vi "write_attributes.vi"(8 "error in (no error)":errorcluster, 10 "attributes":T1, 11 "LinearSVC in":refnum<class "LinearSVC.lvclass">) -> (0 "error out":errorcluster, 3 "LinearSVC out":refnum<class "LinearSVC.lvclass">)   [LabVIEW 2020, in "LinearSVC.lvclass"]
uses:
  LinearSVC.lvclass
  Controls/linear_svc_attributes.ctl
  LinearSVC.lvclass/LinearSVC.ctl
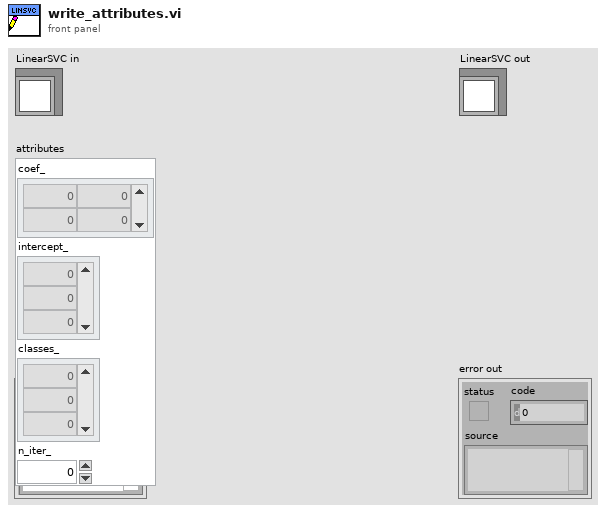
[diagram p1: front panel]
types:
  T1 = typedef "linear_svc_attributes.ctl" = cluster{"coef_":dbl[][], "intercept_":dbl[], "classes_":dbl[], "n_iter_":dbl}
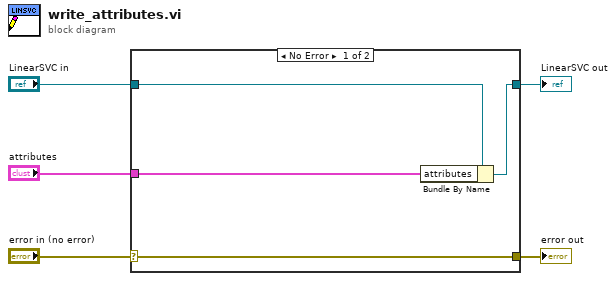
[diagram p0: block diagram]
diagram:
  n1 = case shown="No Error" "error in (no error)" {
    selector: "error in (no error)" -> [w9 w10]
    tunnel: [w9 w10] -> w4
    tunnel: [w7 w11] -> w2
    tunnel: "LinearSVC in" -> [w8 w11]
    tunnel: "attributes" -> [w6 _]
    frame No Error {
      n2 = Bundle By Name(cluster=w8, "attributes"=w6) -> (w7:refnum<class "LinearSVC.lvclass">)
    }
    frame Error {
    }
  }
  "error out" <- w4
  "LinearSVC out" <- w2
